vi "Duplicate Test Executive.vi"(8 "error in (no error)":errorcluster, 11 "Test Executive Ref":refnum<data-value>) -> (0 "error out":errorcluster, 3 "Test Executive Ref out":refnum<data-value>, 5 "Test ID out":string)   [LabVIEW 2017, in "Test Executive.lvlib" / "TestExecutive Ref.lvclass"]
uses:
  <vilib>/gpm_packages/@cs/test-executive/Source/Test Executive/TestExecutive Ref/TestExecutive Ref.lvclass
  <vilib>/gpm_packages/@cs/test-executive/Source/Test Executive/ITestExecutive/ITest Executive.lvclass
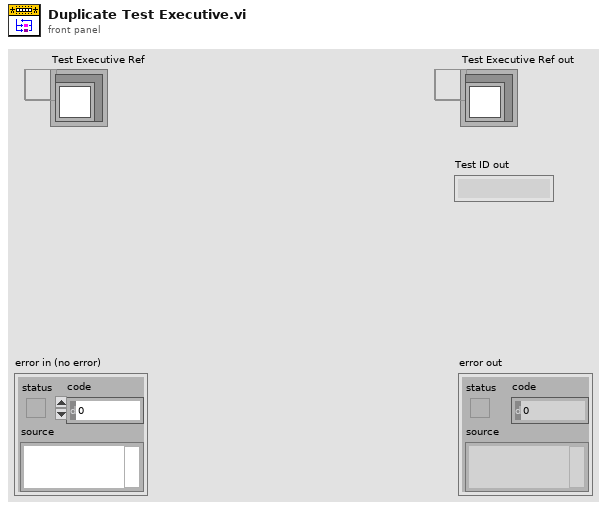
[diagram p1: front panel]
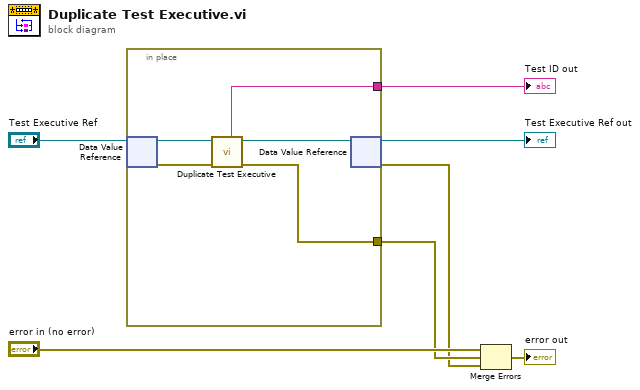
[diagram p0: block diagram]
diagram:
  n1 = in-place {
    in-place-border: [w9] -> w4
    in-place-border: [w8] -> w1
    n2 = in-place-dvr #1("Test Executive Ref") -> (w12:refnum<class "ITest Executive.lvclass">, w11:errorcluster)
    n3 = call-dynamic "Duplicate Test Executive.vi"("error in (no error)"=w11, "ITest Executive in"=w12) -> ("error out"=w9:errorcluster, "ITest Executive out"=w10:refnum<class "ITest Executive.lvclass">, "Test ID out"=w8:string)  [unwired: 7 in]
    n4 = in-place-dvr #1(w10) -> (→"Test Executive Ref out":refnum<data-value>, w3:errorcluster)
  }
  "Test ID out" <- w1
  n5 = Merge Errors("error in (no error)", w4, w3) -> (→"error out":errorcluster)
